vi "数据查询_报警信息.vi"() -> ()   [LabVIEW 2016, in "数据查询.lvlib"]
uses:
  <vilib>/Utility/miscctls.llb/LVPointTypeDef.ctl
  <vilib>/Utility/miscctls.llb/LVRowAndColumnUnsignedTypeDef.ctl
  <userlib>/_OpenG.lib/array/array.llb/Sort 2D Array (String)__ogtk.vi
  <userlib>/_LVST/sqlite_api/Core/Tables/SQLite_List Columns.vi
  <vilib>/addons/database/_DB Variant To Data/Database Variant To Data.xnode
panel:
  in  "列表框":i32(listbox)
  in  "页":i32 format="第%.0f页"
  in  "每页条数":i32=1000
  in  "向后按钮":bool
  in  "向前按钮":bool
  in  "导出":bool
  in  "查询":bool
  out "数据表":string[][](table)
  in  "结束日期":string="2050/01/01"
  in  "起始日期":string="2010/01/01"
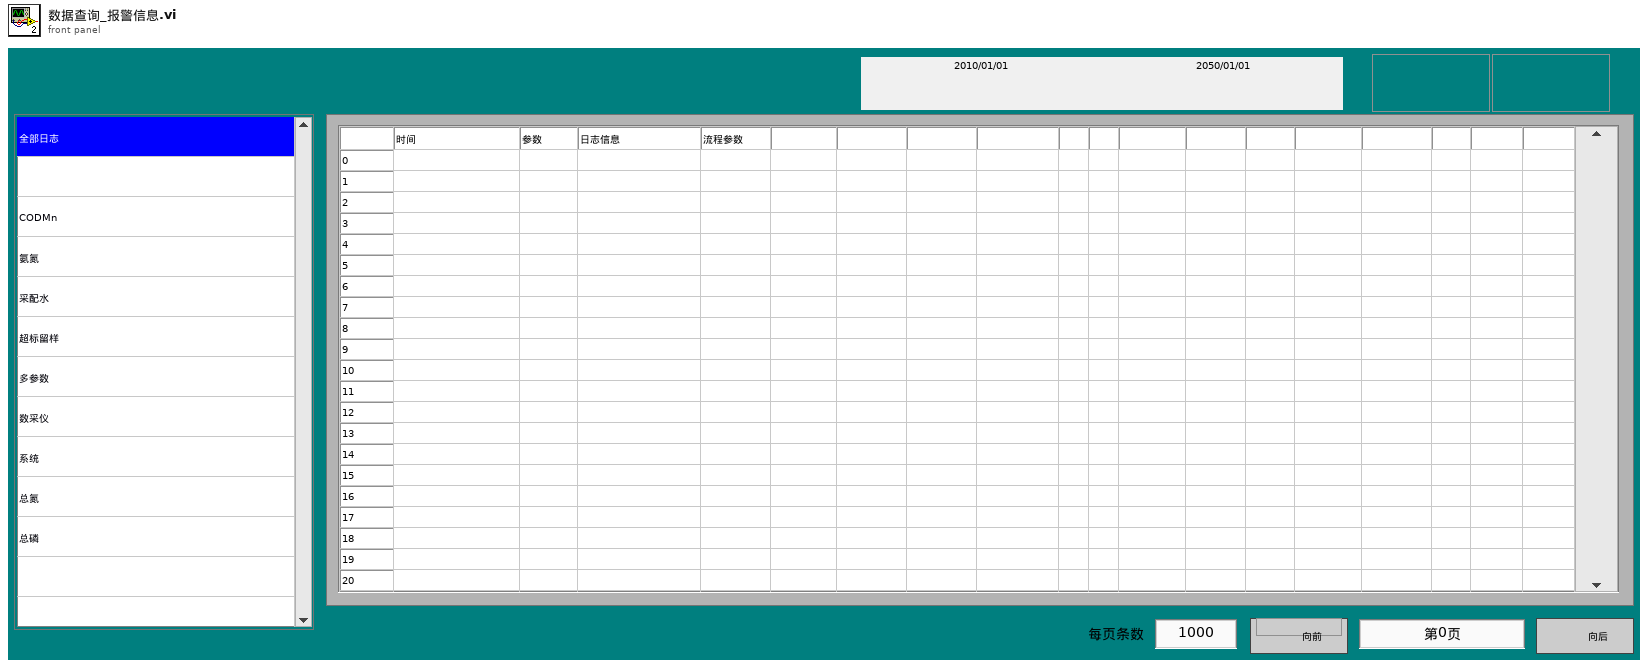
[diagram p1: front panel]
types:
  T1 = typedef "LVPointTypeDef.ctl" = cluster{"Horizontal":i16, "Vertical":i16}
  T2 = typedef "LVDateTimeRec.ctl" = cluster{"秒数的小数部分":dbl, "秒":i32, "分":i32, "时":i32, "日":i32, "月":i32, "年":i32, "天数（周）":i32, "天数（年）":i32, "DST":i32}
  T3 = typedef "数据查询菜单.xctl/数据 1.ctl" = enum32{"数据查询", "仪器数据", "仪器日志", "报警信息", "校准日志"}
  T4 = typedef "数据库类型.ctl" = enum16{"Access", "SQLite"}
  T5 = enum8{"Enabled", "Disabled", "Disabled and Grayed Out"}
  T6 = typedef "LVRowAndColumnUnsignedTypeDef.ctl" = cluster{"Row":u32, "Column":u32}
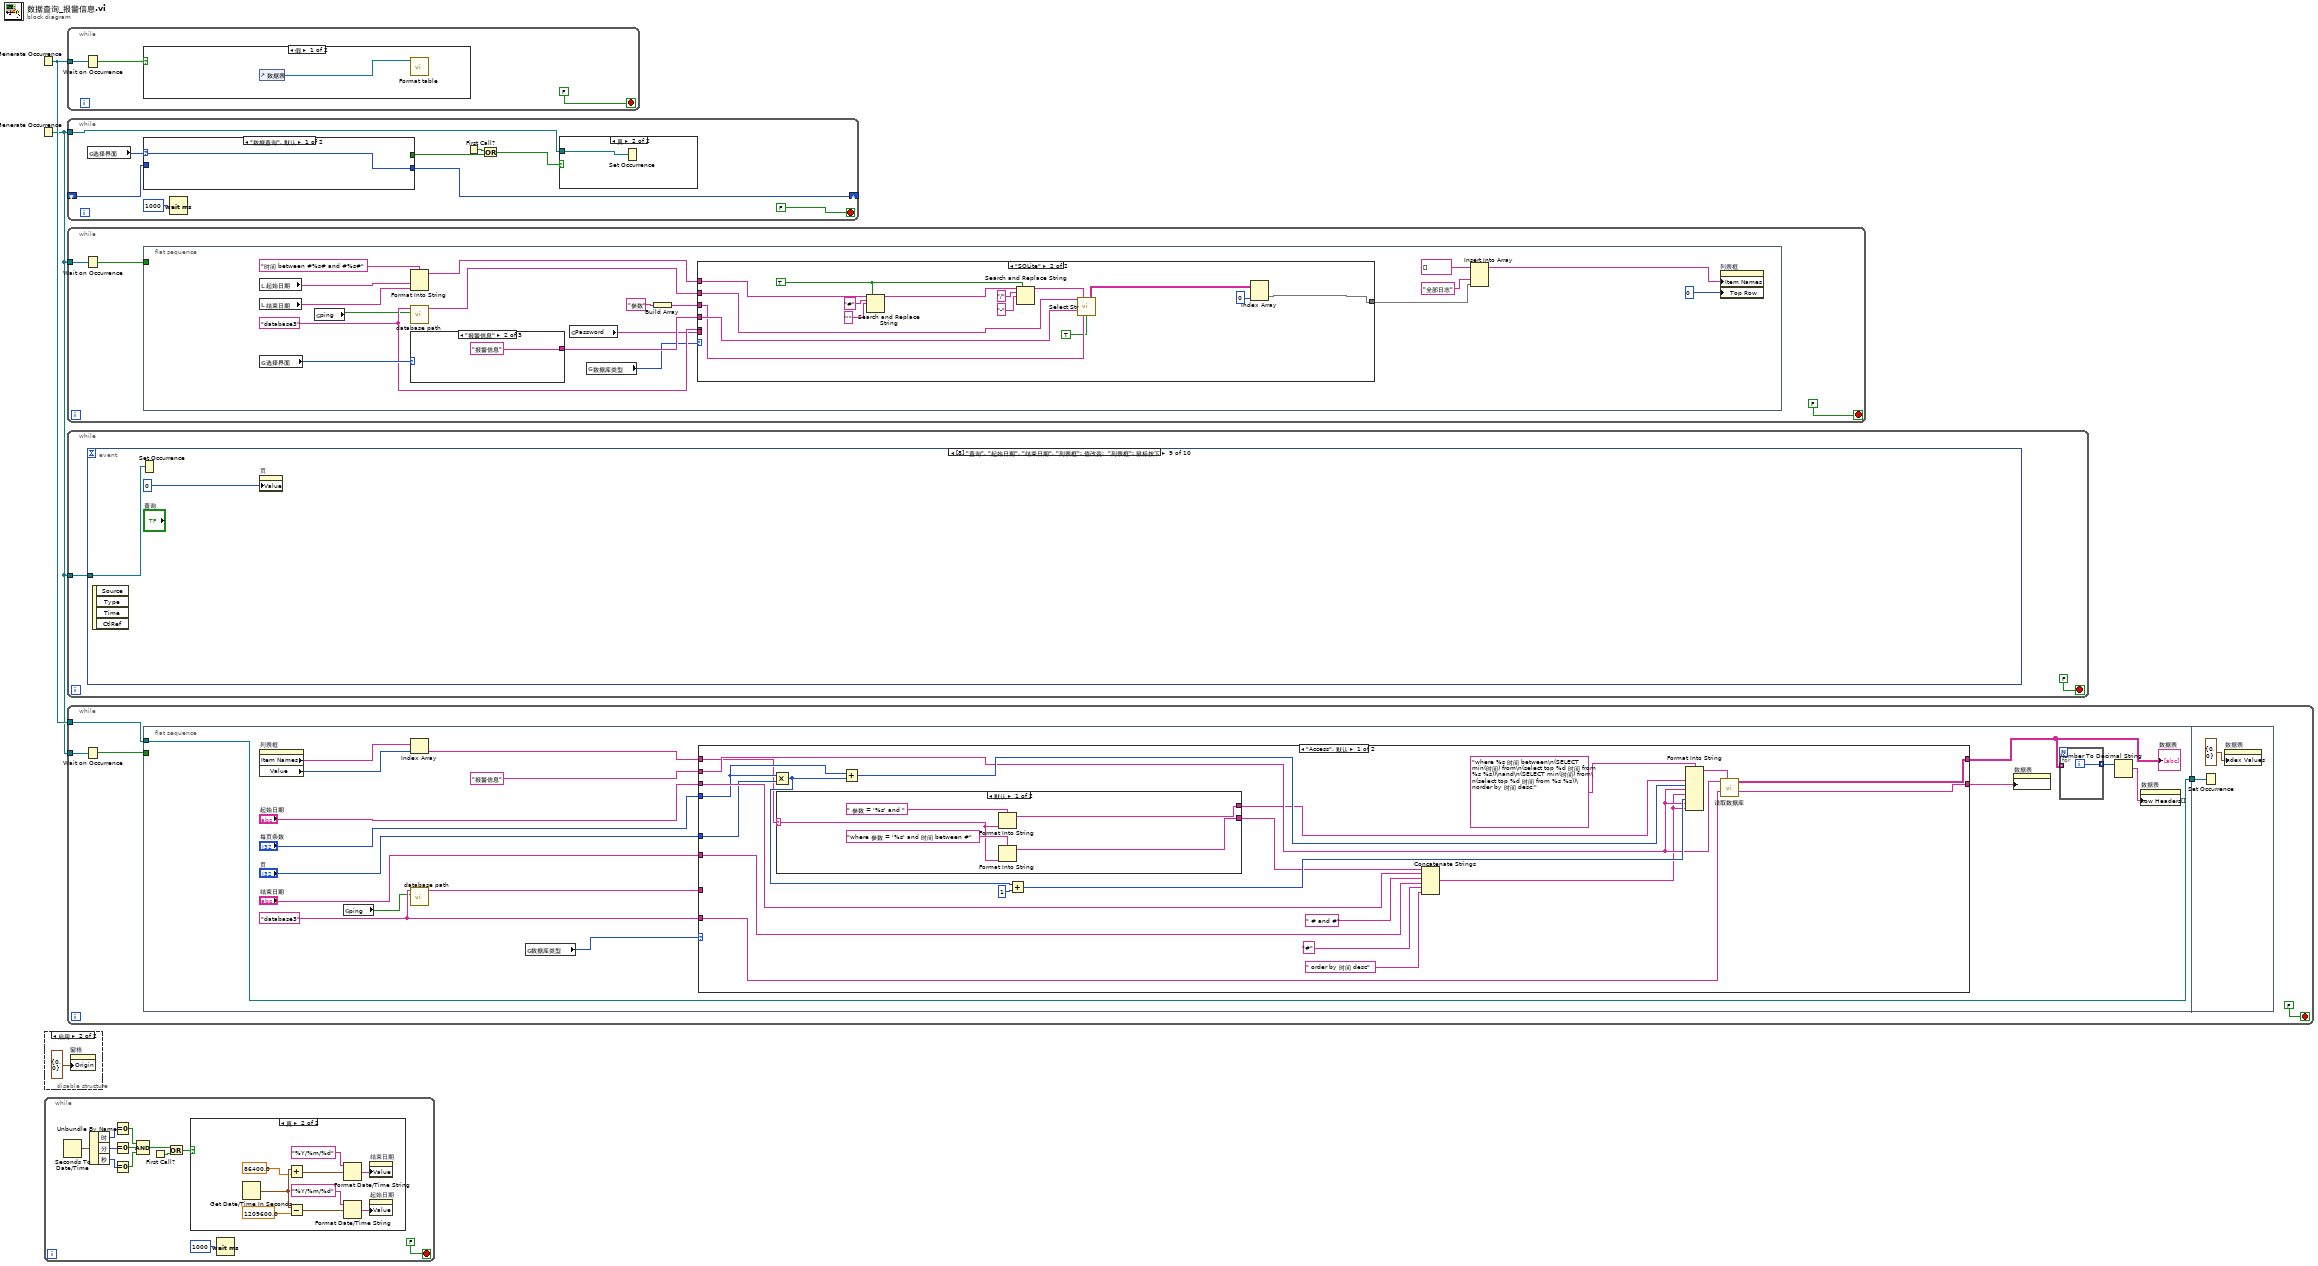
[diagram p0: block diagram]
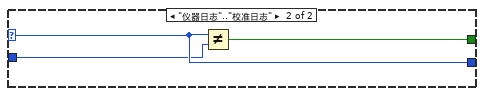
[diagram p3: hidden frame]
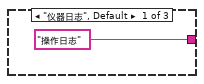
[diagram p5: hidden frame]
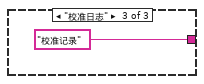
[diagram p6: hidden frame]
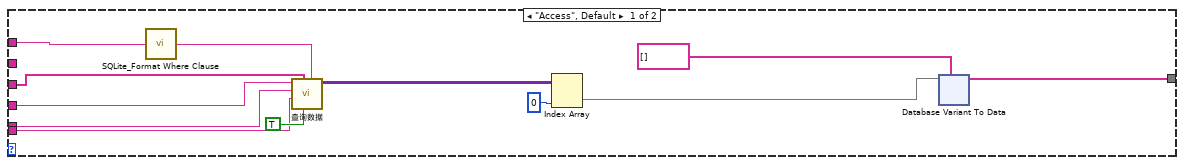
[diagram p7: hidden frame]
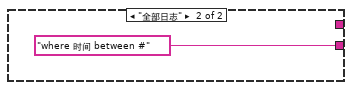
[diagram p8: hidden frame]
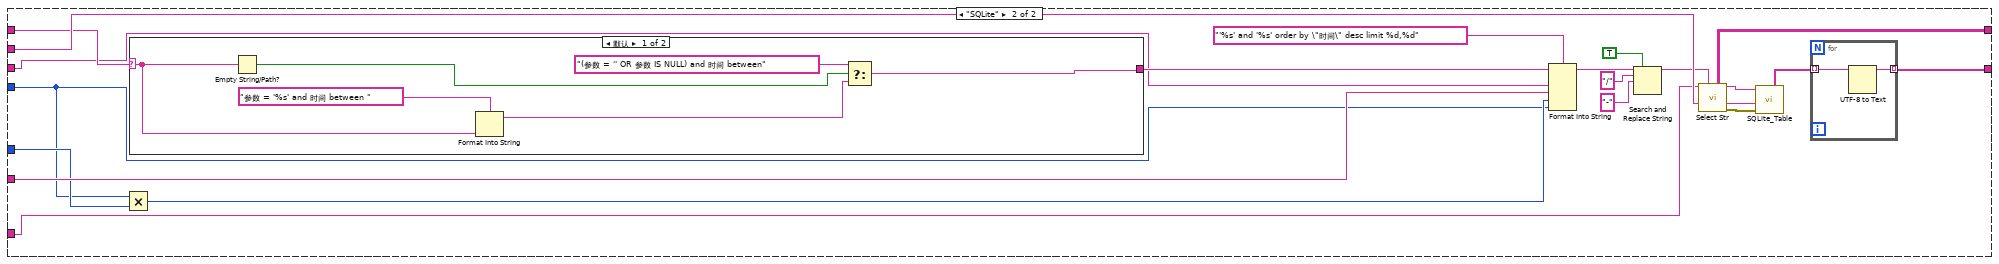
[diagram p9: hidden frame]
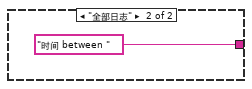
[diagram p10: hidden frame]
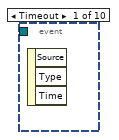
[diagram p12: hidden frame]
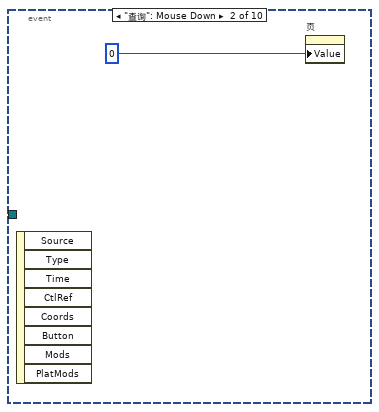
[diagram p13: hidden frame]
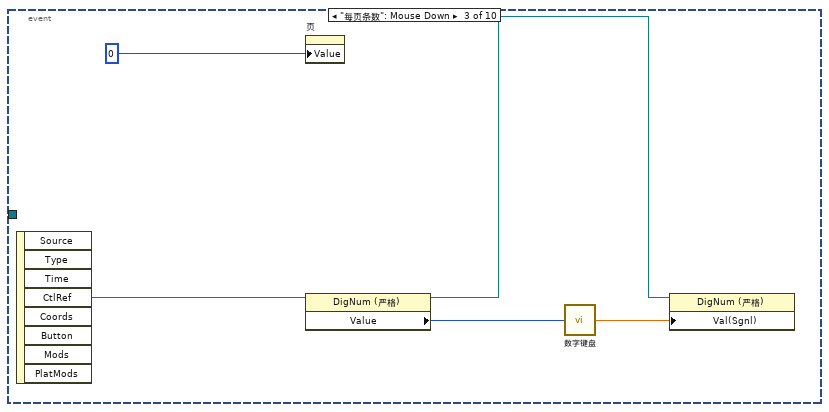
[diagram p14: hidden frame]
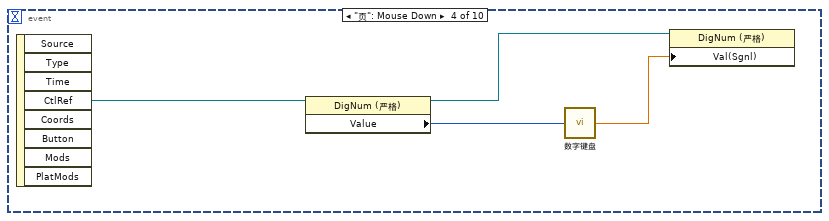
[diagram p15: hidden frame]
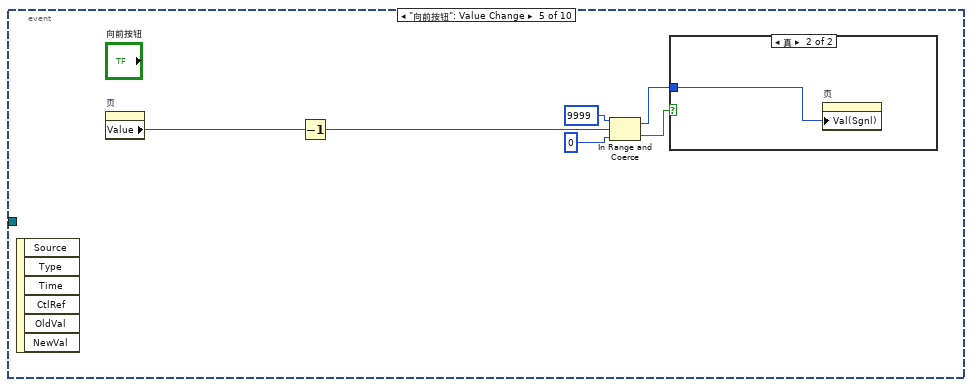
[diagram p16: hidden frame]
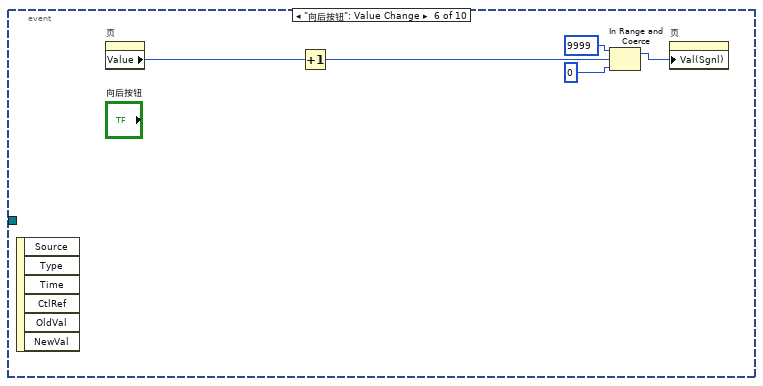
[diagram p18: hidden frame]
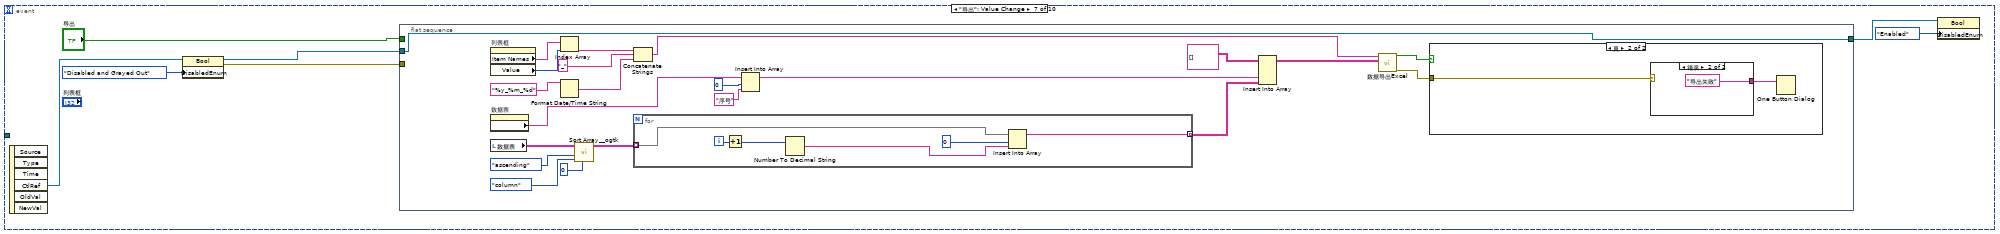
[diagram p19: hidden frame]
diagram:
  n1 = Generate Occurrence() -> (w2:refnum<k4>)
  n2 = Generate Occurrence() -> (w1:refnum<k4>)
  n3 = disable-structure shown="启用" {
    frame Disabled {
    }
    frame Enabled {
      n4 = property on="窗格" class="Pane"("Origin"=T1 {"Horizontal"=0, "Vertical"=0} ("原点")) -> ()  [unwired: 2 in, 2 out]
    }
  }
  n5 = while {
    stop <- FALSE stop-if-true
    n6 = Seconds To Date/Time() -> (date time rec=w15:T2)  [unwired: 2 in]
    n7 = Unbundle By Name(w15) -> ("时"=w14:i32, "分"=w13:i32, "秒"=w12:i32)
    n8 = Equal To 0?(x=w14) -> (x = 0?=w11:bool)
    n9 = Equal To 0?(x=w13) -> (x = 0?=w10:bool)
    n10 = Equal To 0?(x=w12) -> (x = 0?=w9:bool)
    n11 = Compound Arithmetic op=AND ("复合运算")(w11, w10, w9) -> (w6:bool)
    n12 = First Call?() -> (First Call?: T/F=w5:bool)
    n13 = Or(x=w6, y=w5) -> (x .or. y?=w4:bool)
    n14 = case shown="真" w4 {
      frame False {
      }
      frame True {
        n15 = Get Date/Time In Seconds() -> (seconds since 1Jan1904=w20:timestamp)
        n16 = Add(x=w20, y=86400.0) -> (x+y=w18:timestamp)
        n17 = Subtract(x=w20, y=1209600.0) -> (x-y=w21:timestamp)
        n18 = Format Date/Time String(time format string (%c)="%Y/%m/%d" ("时间格式字符串(%c)"), seconds (now)=w18) -> (date/time string=w17:string)  [unwired: 1 in]
        n19 = Format Date/Time String(time format string (%c)="%Y/%m/%d" ("时间格式字符串(%c)"), seconds (now)=w21) -> (date/time string=w23:string)  [unwired: 1 in]
        n20 = property on="结束日期" class="Str"("Value"=w17) -> ()  [unwired: 2 in, 2 out]
        n21 = property on="起始日期" class="Str"("Value"=w23) -> ()  [unwired: 2 in, 2 out]
      }
    }
    n22 = Wait (ms)(milliseconds to wait=u32 1000 ("等待时间（毫秒）")) -> ()  [unwired: 1 out]
  }
  n23 = while {
    tunnel: w2 -> [w25]
    stop <- FALSE stop-if-true
    n24 = Wait on Occurrence(2:w25) -> (0:w27:bool)  [unwired: 2 in]
    n25 = case shown="假" w27 {
      frame False {
        n26 = control-ref of="数据表"() -> (w28:refnum<vi>)
        n27 = call "Format table.vi"("Table输入"=w28) -> ()  [unwired: 11 in]
      }
      frame True {
      }
    }
  }
  n28 = while {
    shift-right: [w34] -> _
    shift-left: _ -> [w33]
    tunnel: w1 -> [w31]
    stop <- FALSE stop-if-true
    n29 = global read "全局变量.vi" "选择界面"() -> (w35:T3)
    n30 = case shown="\"数据查询\", 默认" w35 {
      selector: w35 -> [w39 w42]
      tunnel: [w39 w42] -> w34
      tunnel: w33 -> [_ w41]
      tunnel: [_ w40] -> w32
      frame "数据查询", Default {
      }
      frame "仪器日志".."校准日志" {
        n31 = Not Equal?(x=w42, y=w41) -> (x != y?=w40:bool)
      }
    }
    n32 = Wait (ms)(milliseconds to wait=u32 1000 ("等待时间（毫秒）")) -> ()  [unwired: 1 out]
    n33 = First Call?() -> (First Call?: T/F=w29:bool)
    n34 = Or(x=w29, y=w32) -> (x .or. y?=w30:bool)
    n35 = case shown="真" w30 {
      tunnel: w31 -> [_ w38]
      frame False {
      }
      frame True {
        n36 = Set Occurrence(w38) -> ()
      }
    }
  }
  n37 = while {
    tunnel: w1 -> [w43]
    stop <- FALSE stop-if-true
    n38 = Wait on Occurrence(2:w43) -> (0:w44:bool)  [unwired: 2 in]
    n39 = flat-sequence {
      tunnel: w44 -> [_]
      frame #0 {
        w50 = "database3" ("database")
        n40 = local read "起始日期"() -> (w59:string)
        n41 = local read "结束日期"() -> (w58:string)
        n42 = global read "全局变量.vi" "选择界面"() -> (w53:T3)
        n43 = global read "全局变量.vi" "ping"() -> (w49:bool)
        n44 = Format Into String(format string="时间 between #%s# and #%s#" ("格式字符串"), w59, w58) -> (resulting string=w55:string)  [unwired: 2 in, 1 out]
        n45 = call "database path.vi"("ping"=w49, "database"=w50) -> ("Path out"=w51:string)  [unwired: 8 in, 1 out]
        n46 = case shown="\"报警信息\"" w53 {
          tunnel: ["操作日志" "报警信息" "校准记录"] -> w52
          frame "仪器日志", Default {
          }
          frame "报警信息" {
          }
          frame "校准日志" {
          }
        }
        n47 = global read "外部调用接口全局变量.vi" "Password"() -> (w46:string)
        n48 = global read "外部调用接口全局变量.vi" "数据库类型"() -> (w47:T4)
        n49 = Build Array("参数") -> (w54:string[])
        n50 = case shown="\"SQLite\"" w47 {
          tunnel: w52 -> [w78 w131]
          tunnel: w54 -> [w77 w130]
          tunnel: [w71 w117] -> w48
          tunnel: w55 -> [w70 w126]
          tunnel: w50 -> [w68 _]
          tunnel: w51 -> [_ w118]
          tunnel: w46 -> [w67 _]
          frame "Access", Default {
            n51 = call <userlib>:"SQLite_Format Where Clause.vi"("Where clause"=w70) -> ("String"=w69:string)  [unwired: 4 in]
            n52 = call "查询数据.vi"("condition"=w69, "Distinct"=TRUE, "columns"=w77, "Password"=w67, "database"=w68, "table"=w78) -> ("data"=w76:variant[][])  [unwired: 4 in, 1 out]
            n53 = Index Array(array=w76, index (col)=0 ("禁用的索引 (列)")) -> (element=w75:variant[])  [unwired: 1 in]
            n54 = xnode "Database Variant To Data"("database variant"=w75, "type"=string[] []) -> ("data"=w71:string[])  [unwired: 1 in, 1 out]
          }
          frame "SQLite" {
            w119 = TRUE ("替换全部？(F)")
            n55 = Search and Replace String(replace all?=w119, input string=w126, search string="#" ("搜索字符串"), replace string="'" ("替换字符串(\"\")")) -> (result string=w121:string)  [unwired: 4 in, 3 out]
            n56 = Search and Replace String(replace all?=w119, input string=w121, search string="/" ("搜索字符串"), replace string="-" ("替换字符串(\"\")")) -> (result string=w120:string)  [unwired: 4 in, 3 out]
            n57 = call "Select Str.vi"("DB Path"=w118, "Where Clause"=w120, "Tables Name"=w131, "Columns"=w130, "Distinct"=TRUE) -> ("Results"=w128:string[][])  [unwired: 7 in, 3 out]
            n58 = Index Array(array=w128, index (col)=0 ("禁用的索引 (列)")) -> (element=w117:string[])  [unwired: 1 in]
          }
        }
        n59 = Insert Into Array(array=string[] [], new element #1="全部日志" ("新元素/子数组"), new element #2=w48) -> (w57:string[])  [unwired: 1 in]
        n60 = property on="列表框" class="LstBox (严格)"("Item Names"=w57, "Top Row"=0 ("顶行")) -> ()  [unwired: 2 in, 2 out]
      }
    }
  }
  n61 = while {
    tunnel: w1 -> [w132]
    stop <- FALSE stop-if-true
    n62 = event shown="[8] \"查询\", \"起始日期\", \"结束日期\", \"列表框\": 值改变;  \"列表框\": 鼠标按下" {
      selector: _ -> [_ _ _ _ _ _ _ _ _ _]
      dyn-events: _ -> [_ _ _ _ _ _ _ _ _ _]
      timeout: _ -> [_ _ _ _ _ _ _ _ _ _]
      tunnel: w132 -> [_ _ _ _ _ _ _ _ w201 w202]
      event Timeout {
        n63 = event-data() -> ()  [unwired: 1 in, 3 out]
      }
      event "查询": Mouse Down {
        n64 = event-data() -> ()  [unwired: 1 in, 8 out]
        n65 = property on="页" class="DigNum (严格)"("Value"=0 ("页")) -> ()  [unwired: 2 in, 2 out]
      }
      event "每页条数": Mouse Down {
        n66 = event-data() -> ("CtlRef"=w139:refnum<vi>)  [unwired: 1 in, 7 out]
        n67 = property on="页" class="DigNum (严格)"("Value"=0 ("页")) -> ()  [unwired: 2 in, 2 out]
        n68 = property class="DigNum (严格)"(reference=w139) -> (reference out=w136:refnum<vi>, "Value"=w138:i32)  [unwired: 1 in, 1 out]
        n69 = call "数字键盘.vi"("OldNumber"=w138) -> ("NewNumber"=w137:sgl)
        n70 = property class="DigNum (严格)"(reference=w136, "Val(Sgnl)"=w137) -> ()  [unwired: 1 in, 2 out]
      }
      event "页": Mouse Down {
        n71 = event-data() -> ("CtlRef"=w143:refnum<vi>)  [unwired: 1 in, 7 out]
        n72 = property class="DigNum (严格)"(reference=w143) -> (reference out=w140:refnum<vi>, "Value"=w142:i32)  [unwired: 1 in, 1 out]
        n73 = call "数字键盘.vi"("OldNumber"=w142) -> ("NewNumber"=w141:sgl)
        n74 = property class="DigNum (严格)"(reference=w140, "Val(Sgnl)"=w141) -> ()  [unwired: 1 in, 2 out]
      }
      event "向前按钮": Value Change {
        n75 = event-data() -> ()  [unwired: 1 in, 6 out]
        n76 = property on="页" class="DigNum (严格)"() -> ("Value"=w149:i32)  [unwired: 2 in, 2 out]
        n77 = Decrement(x=w149) -> (x-1=w148:i32)
        n78 = In Range and Coerce(upper limit=9999 ("上限"), x=w148, lower limit=0 ("下限")) -> (coerced(x)=w145:i32, In Range?=w144:bool)
        n79 = case shown="真" w144 {
          tunnel: w145 -> [_ w150]
          frame False {
          }
          frame True {
            n80 = property on="页" class="DigNum (严格)"("Val(Sgnl)"=w150) -> ()  [unwired: 2 in, 2 out]
          }
        }
      }
      event "向后按钮": Value Change {
        n81 = event-data() -> ()  [unwired: 1 in, 6 out]
        n82 = property on="页" class="DigNum (严格)"() -> ("Value"=w155:i32)  [unwired: 2 in, 2 out]
        n83 = Increment(x=w155) -> (x+1=w154:i32)
        n84 = In Range and Coerce(upper limit=u32 9999 ("上限"), x=w154, lower limit=u32 0 ("下限")) -> (coerced(x)=w151:u32)  [unwired: 1 out]
        n85 = property on="页" class="DigNum (严格)"("Val(Sgnl)"=w151) -> ()  [unwired: 2 in, 2 out]
      }
      event "导出": Value Change {
        n86 = event-data() -> ("CtlRef"=w156:refnum<vi>)  [unwired: 1 in, 5 out]
        n87 = property class="Bool"(reference=w156, "DisabledEnum"=T5."Disabled and Grayed Out" ("禁用")) -> (reference out=w160:refnum<vi>, error out=w161:errorcluster)  [unwired: 1 in]
        n88 = flat-sequence {
          tunnel: w161 -> [_]
          tunnel: [w180] -> w159
          tunnel: w160 -> [w180]
          tunnel: "导出" -> [_]
          frame #0 {
            n89 = property on="列表框" class="LstBox (严格)"() -> ("Item Names"=w165:string[], "Value"=w164:i32)  [unwired: 2 in, 2 out]
            n90 = property on="数据表" class="Tbl (严格)"() -> ("Column Headers[]"=w173:string[])  [unwired: 2 in, 2 out]
            n91 = local read "数据表"() -> (w184:string[][])
            n92 = Index Array(array=w165, index=w164) -> (element=w163:string)
            n93 = Format Date/Time String(time format string (%c)="%y_%m_%d" ("时间格式字符串(%c)")) -> (date/time string=w177:string)  [unwired: 2 in]
            n94 = call-poly <userlib>:"Sort Array__ogtk.vi"("Column/Row to Sort By"=u32 0, "Sort By in"=enum16{"row", "column"}."column", "Order"=enum16{"ascending", "descending"}."ascending", "Array in"=w184) -> ("Sorted Array out"=w166:string[][])  [unwired: 4 in, 3 out]
            n95 = Concatenate Strings(w163, "_" ("字符串"), w177) -> (w175:string)
            n96 = for {
              tunnel: w166 -> [w193] mode=indexing
              tunnel: [w192] -> w170 mode=indexing
              i -> [w194]
              n97 = Increment(x=w194) -> (x+1=w190:i32)
              n98 = Number To Decimal String(number=w190) -> (decimal integer string=w189:string)  [unwired: 1 in]
              n99 = Insert Into Array(array=w193, index=0 ("索引"), new element=w189) -> (w192:string[])
            }
            n100 = Insert Into Array(array=w173, index=0 ("索引"), new element="序号" ("新元素/子数组")) -> (w174:string[])
            n101 = Insert Into Array(array=string[][] [], new element #1=w174, new element #2=w170) -> (w169:string[][])  [unwired: 2 in]
            n102 = call "数据导出Excel.vi"("text data"=w169, "default name"=w175) -> ("error out"=w168:errorcluster, "布尔"=w167:bool)  [unwired: 8 in]
            n103 = case shown="真" w167 {
              tunnel: w168 -> [_ w186]
              frame False {
              }
              frame True {
                n104 = case shown="错误" w186 {
                  tunnel: ["导出成功" ("消息") "导出失败" ("消息")] -> w185
                  frame No Error {
                  }
                  frame Error {
                  }
                }
                n105 = One Button Dialog(message=w185) -> ()  [unwired: 1 in, 1 out]
              }
            }
          }
        }
        n106 = property class="Bool"(reference=w159, "DisabledEnum"=T5."Enabled" ("禁用")) -> ()  [unwired: 1 in, 2 out]
      }
      event "起始日期", "结束日期": Mouse Down {
        n107 = event-data() -> ("CtlRef"=w199:refnum<vi>)  [unwired: 1 in, 7 out]
        n108 = property on="页" class="DigNum (严格)"("Value"=0 ("页")) -> ()  [unwired: 2 in, 2 out]
        n109 = property class="Str"(reference=w199) -> (reference out=w197:refnum<vi>, "Value"=w198:string)  [unwired: 1 in, 1 out]
        n110 = call "日期键盘.vi"("原值"=w198) -> ("x+y"=w196:string)  [unwired: 10 in]
        n111 = property class="Str"(reference=w197, "Val(Sgnl)"=w196) -> ()  [unwired: 1 in, 2 out]
      }
      event "查询", "起始日期", "结束日期", "列表框": Value Change; "列表框": Mouse Down {
        n112 = event-data() -> ()  [unwired: 1 in, 4 out]
        n113 = Set Occurrence(w201) -> ()
        n114 = property on="页" class="DigNum (严格)"("Value"=0 ("页")) -> ()  [unwired: 2 in, 2 out]
      }
      event "页", "每页条数": Value Change {
        n115 = event-data() -> ()  [unwired: 1 in, 6 out]
        n116 = Set Occurrence(w202) -> ()
      }
    }
  }
  n117 = while {
    tunnel: w1 -> [w206]
    tunnel: w2 -> [w203]
    stop <- FALSE stop-if-true
    n118 = Wait on Occurrence(2:w206) -> (0:w205:bool)  [unwired: 2 in]
    n119 = flat-sequence {
      tunnel: w205 -> [_]
      tunnel: [w220] -> w204
      tunnel: w203 -> [w220]
      tunnel: w204 -> [w283]
      frame #0 {
        w210 = "database3" ("database")
        n120 = property on="列表框" class="LstBox (严格)"() -> ("Item Names"=w221:string[], "Value"=w222:i32)  [unwired: 2 in, 2 out]
        n121 = global read "全局变量.vi" "ping"() -> (w209:bool)
        n122 = Index Array(array=w221, index=w222) -> (element=w217:string)
        n123 = call "database path.vi"("ping"=w209, "database"=w210) -> ("Path out"=w211:string)  [unwired: 8 in, 1 out]
        n124 = global read "外部调用接口全局变量.vi" "数据库类型"() -> (w208:T4)
        n125 = case shown="\"Access\", 默认" w208 {
          tunnel: "起始日期" -> [w245 w264]
          tunnel: "结束日期" -> [w244 w263]
          tunnel: [w241 w253] -> w219
          tunnel: [w239 w268] -> w218
          tunnel: "每页条数" -> [w233 w255]
          tunnel: "页" -> [w232 w257]
          tunnel: "报警信息" -> [w231 w272]
          tunnel: w210 -> [w229 _]
          tunnel: w217 -> [w227 w267]
          tunnel: w211 -> [_ w252]
          frame "Access", Default {
            n126 = Multiply(x=w233, y=w232) -> (x*y=w237:i32)
            n127 = case shown="默认" w227 {
              selector: w227 -> [w247 _]
              tunnel: [w250 "where 时间 between #" ("condition")] -> w225
              tunnel: [w246 _] -> w226
              frame Default {
                n128 = Format Into String(format string=" 参数 = '%s' and " ("condition"), w247) -> (resulting string=w246:string)  [unwired: 2 in, 1 out]
                n129 = Format Into String(format string="where 参数 = '%s' and 时间 between #" ("condition"), w247) -> (resulting string=w250:string)  [unwired: 2 in, 1 out]
              }
              frame "全部日志" {
              }
            }
            n130 = Add(x=w233, y=w237) -> (x+y=w235:i32)
            n131 = Add(x=w237, y=u32 1) -> (x+y=w234:u32)
            n132 = Concatenate Strings(w225, w245, " # and #" ("condition"), w244, "#" ("condition"), " order by 时间 desc" ("字符串")) -> (w230:string)
            n133 = Format Into String(format string="where %s 时间 between\n(SELECT min(时间) from\n(select top %d 时间 from %s %s))\nand\n(SELECT min(时间) from\n(select top %d 时间 from %s %s))\norder by 时间 desc;" ("格式字符串"), w226, w235, w231, w230, w234, w231, w230) -> (resulting string=w228:string)  [unwired: 2 in, 1 out]
            n134 = call "读取数据库.vi"("condition"=w228, "database"=w229, "组合框"=w231) -> ("columns"=w241:string[], "表格"=w239:string[][])  [unwired: 5 in, 2 out]
          }
          frame "SQLite" {
            n135 = Multiply(x=w255, y=w257) -> (x*y=w256:i32)
            n136 = case shown="默认" w267 {
              selector: w267 -> [w275 _]
              tunnel: [w276 "时间 between " ("condition")] -> w266
              frame Default {
                n137 = Empty String/Path?(string/path=w275) -> (empty?=w280:bool)
                n138 = Format Into String(format string="参数 = '%s' and 时间 between " ("condition"), w275) -> (resulting string=w277:string)  [unwired: 2 in, 1 out]
                n139 = Select(t="(参数 = '' OR 参数 IS NULL) and 时间 between" ("condition"), s=w280, f=w277) -> (s? t:f=w276:string)
              }
              frame "全部日志" {
              }
            }
            n140 = Format Into String(format string="'%s' and '%s' order by \"时间\" desc limit %d,%d" ("格式字符串"), initial string=w266, w264, w263, w256, w255) -> (resulting string=w260:string)  [unwired: 1 in, 1 out]
            n141 = Search and Replace String(replace all?=TRUE ("替换全部？(F)"), input string=w260, search string="/" ("搜索字符串"), replace string="-" ("替换字符串(\"\")")) -> (result string=w259:string)  [unwired: 4 in, 3 out]
            n142 = call "Select Str.vi"("DB Path"=w252, "Where Clause"=w259, "Tables Name"=w272) -> ("Results"=w268:string[][], "DB Path Out"=w271:string, "Table Name Out"=w270:string, "error out"=w269:errorcluster)  [unwired: 9 in]
            n143 = call-poly <userlib>:"SQLite_Table.vi"("DB Path"=w271, "Table Name"=w270, "error in (no error)"=w269) -> ("Columns"=w254:string[])  [unwired: 4 in, 3 out]
            n144 = for {
              tunnel: w254 -> [w274] mode=indexing
              tunnel: [w273] -> w253 mode=indexing
              n145 = UTF-8 to Text(11:w274) -> (3:w273:string)  [unwired: 2 in, 1 out]
            }
          }
        }
        "数据表" <- w218
        n146 = property on="数据表" class="Tbl (严格)"("Column Headers[]"=w219) -> ()  [unwired: 2 in, 2 out]
        n147 = for {
          tunnel: [w282] -> w224 mode=indexing
          tunnel: w218 -> [_] mode=indexing
          i -> [w282]
        }
        n148 = Number To Decimal String(number=w224) -> (decimal integer string=w223:string[])  [unwired: 1 in]
        n149 = property on="数据表" class="Tbl (严格)"("Row Headers[]"=w223) -> ()  [unwired: 2 in, 2 out]
      }
      frame #1 {
        n150 = Set Occurrence(w283) -> ()
        n151 = property on="数据表" class="Tbl (严格)"("Index Values"=T6 {"Row"=0, "Column"=0} ("索引值")) -> ()  [unwired: 2 in, 2 out]
      }
    }
  }
